vi "NT to XML Boolean.vi"(10 "NT Name":string="Boolean", 11 "Subsytem XML Name":path) -> (2 "Global Value":bool)   [LabVIEW 2020]
uses:
  <vilib>/Rock Robotics/Network Tables/NT Read Boolean.vi
  <vilib>/Utility/xml.llb/Write to XML File(string).vi
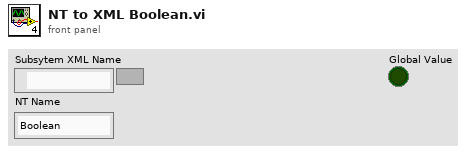
[diagram p1: front panel]
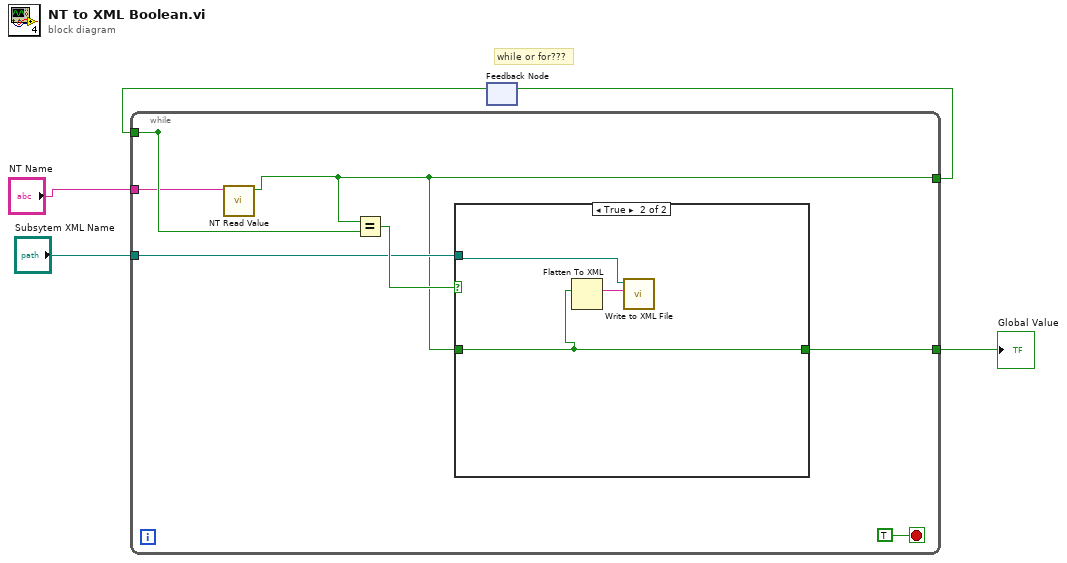
[diagram p0: block diagram]
diagram:
  # "while or for???"
  n1 = feedback #1() -> (w4:bool)  [unwired: 1 in]
  n2 = while {
    tunnel: [w6] -> w5
    tunnel: [w12] -> _
    tunnel: w4 -> [w12]
    tunnel: "Subsytem XML Name" -> [w9]
    tunnel: "NT Name" -> [w8]
    tunnel: [w7] -> w1
    stop <- TRUE stop-if-true
    n3 = call-poly <vilib>:"NT Read Value.vi"("Name"=w8) -> ("Boolean"=w6:bool)  [unwired: 9 in, 1 out]
    n4 = Equal?(x=w6, y=w12) -> (x = y?=w11:bool)
    n5 = case shown="True" w11 {
      tunnel: w9 -> [_ w15]
      tunnel: [w13 w14] -> w7
      tunnel: w6 -> [w13 w14]
      frame False {
      }
      frame True {
        n6 = Flatten To XML(anything=w14) -> (xml string=w16:string)
        n7 = call-poly <vilib>:"Write to XML File.vi"("XML Input"=w16, "XML File Path"=w15) -> ()  [unwired: 7 in, 3 out]
      }
    }
  }
  "Global Value" <- w1
  n8 = feedback-in #1(w5) -> ()
